vi "624WPI_CameraRead MJPG for Dashboard.vi"(6 "Camera Settings":T2={"fps"=30, "compression"=30, "Image Size"=enum."320x240", "Config Shown"=FALSE}, 7 "USB Cam TCP Port":u16=1180, 8 "Rec Mode":u16(ring) items=["O", "*", "Open Playback Panel"], 9 "Camera IP":string, 10 "Camera Mode":u16(ring) items=["Camera Off", "USB Camera SW", "USB Camera HW", "IP Camera"], 11 "Refnum in":T1) -> (2 "Active":bool, 3 "Refnum out":T1, 4 "FPS":dbl, 5 "Bandwidth (Mbps)":dbl)   [LabVIEW 2016]
uses:
  <vilib>/Rock Robotics/WPI/Camera/WPI_CameraSettings Read MJPG.ctl
  <vilib>/Rock Robotics/WPI/Camera/WPI_CameraImageSize.ctl
  <vilib>/vision/Image Controls.llb/IMAQ Image.ctl
  <vilib>/Rock Robotics/WPI/Dashboard/WPI_DashboardLogging Global.vi
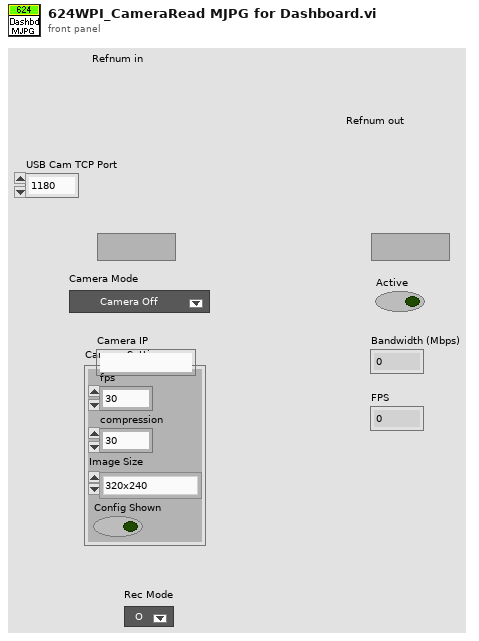
[diagram p1: front panel]
types:
  T1 = typedef "IMAQ Image.ctl" = refnum<image>
  T2 = typedef "WPI_CameraSettings Read MJPG.ctl" = cluster{"fps":i32, "compression":i32, "Image Size":T3, "Config Shown":bool}
  T3 = typedef "WPI_CameraImageSize.ctl" = enum16{"640x480", "320x240", "160x120", "Custom"}
  T4 = typedef "IMAQ AVI2 Refnum.ctl" = refnum<k20>
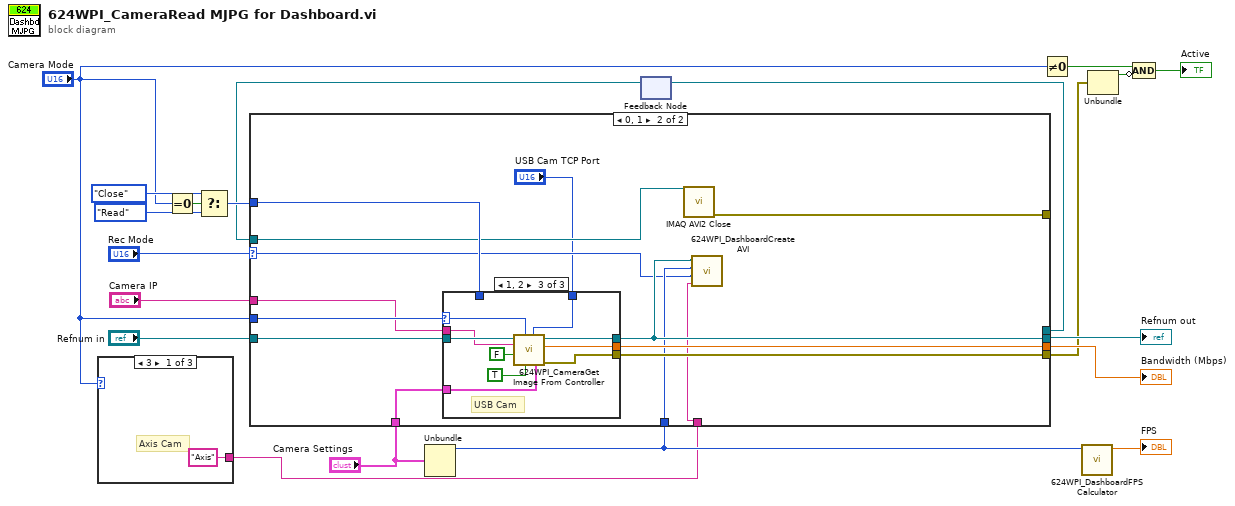
[diagram p0: block diagram]
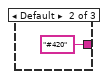
[diagram p2: hidden frame]
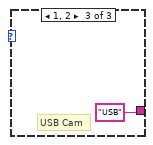
[diagram p3: hidden frame]
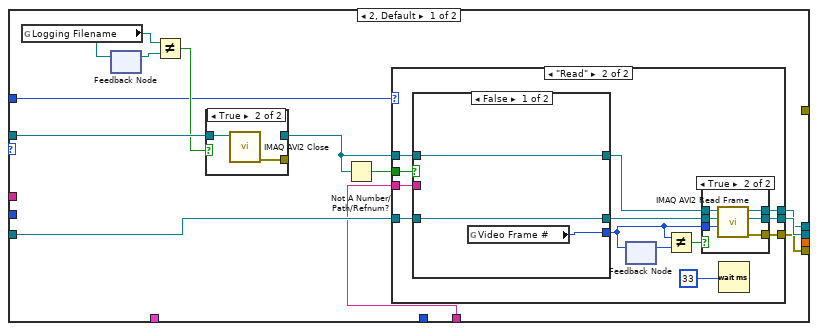
[diagram p4: hidden frame]
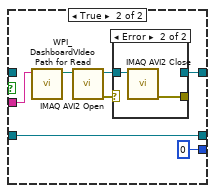
[diagram p7: hidden frame]
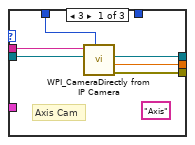
[diagram p10: hidden frame]
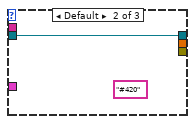
[diagram p11: hidden frame]
diagram:
  n1 = case shown="3" "Camera Mode" {
    tunnel: ["Axis" "#420" "USB"] -> w1
    frame 3 {
      # "Axis Cam"
    }
    frame Default {
    }
    frame 1, 2 {
      # "USB Cam"
    }
  }
  n2 = Equal To 0?(x="Camera Mode") -> (x = 0?=w6:bool)
  n3 = Select(t=enum16{"Read", "Reopen", "Close"}."Close" ("Operation"), s=w6, f=enum16{"Read", "Reopen", "Close"}."Read" ("Operation")) -> (s? t:f=w17:enum16{"Read", "Reopen", "Close"})
  n4 = Unbundle("Camera Settings") -> ("fps"=w4:i32)  [unwired: 3 out]
  n5 = feedback #1() -> (w9:T4)  [unwired: 1 in]
  n6 = case shown="0, 1" "Rec Mode" {
    selector: "Rec Mode" -> [_ w78]
    tunnel: "Camera Settings" -> [_ w88]
    tunnel: w17 -> [w25 w87]
    tunnel: [_ w86] -> w14
    tunnel: [w35 w80] -> w10
    tunnel: "Refnum in" -> [w33 w85]
    tunnel: "Camera IP" -> [_ w77]
    tunnel: w4 -> [_ w79]
    tunnel: w9 -> [w29 w83]
    tunnel: [w32 _] -> w8
    tunnel: [w31 w84] -> w7
    tunnel: [_ w82] -> _
    tunnel: "Camera Mode" -> [_ w81]
    tunnel: w1 -> [w24 w75]
    frame 2, Default {
      n7 = global read "WPI_DashboardLogging Global.vi" "Logging Filename"() -> (w28:path)
      n8 = feedback #2() -> (w27:path)  [unwired: 1 in]
      n9 = feedback-in #2(w28) -> ()
      n10 = Not Equal?(x=w28, y=w27) -> (x != y?=w26:bool)
      n11 = case shown="True" w26 {
        tunnel: [w72 _] -> w30
        tunnel: w29 -> [w72 w74]
        tunnel: [_ w73] -> _
        frame False {
        }
        frame True {
          n12 = call "IMAQ AVI2 Close"("AVI Refnum"=w74) -> ("error out"=w73:errorcluster)  [unwired: 10 in]
        }
      }
      n13 = Not A Number/Path/Refnum?(number/path/refnum=w30) -> (NaN/Path/Refnum?=w34:bool)
      n14 = case shown="\"Read\"" w25 {
        tunnel: [w36 w50] -> w35
        tunnel: w34 -> [_ w49]
        tunnel: w33 -> [w36 w46]
        tunnel: [w37 w45] -> w32
        tunnel: [_ w44] -> w31
        tunnel: w24 -> [_ w43]
        tunnel: w30 -> [w37 w42]
        frame "Close", Default {
        }
        frame "Read" {
          n15 = case shown="False" w49 {
            tunnel: [w61 w66] -> w48
            tunnel: w42 -> [w61 _]
            tunnel: [w60 w68] -> w47
            tunnel: w46 -> [w60 w68]
            tunnel: [w59 0 ("Video Frame #")] -> w39
            tunnel: w43 -> [_ w63]
            frame False {
              n16 = global read "WPI_DashboardLogging Global.vi" "Video Frame #"() -> (w59:i32)
            }
            frame True {
              n17 = call <vilib>:"WPI_DashboardVIdeo Path for Read.vi"("Camera IP"=w63) -> ("Video Path"=w62:path)  [unwired: 10 in]
              n18 = call "IMAQ AVI2 Open"("AVI File Path"=w62) -> ("error out"=w67:errorcluster, "AVI Refnum"=w65:T4)  [unwired: 9 in]
              n19 = case shown="Error" w67 {
                tunnel: [w69 _] -> w66
                tunnel: w65 -> [w69 w71]
                tunnel: [_ w70] -> _
                frame No Error {
                }
                frame Error {
                  n20 = call "IMAQ AVI2 Close"("AVI Refnum"=w71) -> ("error out"=w70:errorcluster)  [unwired: 10 in]
                }
              }
            }
          }
          n21 = feedback #3() -> (w40:i32)  [unwired: 1 in]
          n22 = feedback-in #3(w39) -> ()
          n23 = Not Equal?(x=w39, y=w40) -> (x != y?=w41:bool)
          n24 = case shown="True" w41 {
            tunnel: [w51 w58] -> w50
            tunnel: w48 -> [w52 w57]
            tunnel: w47 -> [w51 w56]
            tunnel: [w52 w55] -> w45
            tunnel: [_ w54] -> w44
            tunnel: w39 -> [_ w53]
            frame False {
            }
            frame True {
              n25 = call "IMAQ AVI2 Read Frame"("Frame Number"=w53, "Image"=w56, "AVI Refnum"=w57) -> ("error out"=w54:errorcluster, "Image Out"=w58:T1, "AVI Refnum (duplicate)"=w55:T4)  [unwired: 6 in]
            }
          }
          n26 = Wait (ms)(milliseconds to wait=33) -> ()  [unwired: 1 out]
        }
      }
    }
    frame 0, 1 {
      n27 = case shown="1, 2" w81 {
        selector: w81 -> [_ _ w98]
        tunnel: w88 -> [_ _ w100]
        tunnel: w87 -> [w89 _ _]
        tunnel: [w93 _ w99] -> w86
        tunnel: w85 -> [w91 w95 w105]
        tunnel: w77 -> [w90 _ w102]
        tunnel: [w94 _ w103] -> w84
        tunnel: [w92 w95 w104] -> w80
        tunnel: "USB Cam TCP Port" -> [_ _ w97]
        frame 3 {
          (unwired) "Axis"
          # "Axis Cam"
          n28 = call <vilib>:"WPI_CameraDirectly from IP Camera.vi"("Operation"=w89, "Image"=w91, "address"=w90) -> ("error out"=w94:errorcluster, "Bandwidth (Mbps)"=w93:dbl, "Image Out"=w92:T1)  [unwired: 6 in]
        }
        frame Default {
          (unwired) "#420"
        }
        frame 1, 2 {
          # "USB Cam"
          n29 = call "624WPI_CameraGet Image From Controller.vi"("Camera Settings"=w100, "port"=w97, "USB"=TRUE, "Camera Mode"=w98, "Close?"=FALSE, "Controller Address"=w102, "Image"=w105) -> ("error out"=w103:errorcluster, "Bandwidth (Mbps)"=w99:dbl, "Image Out"=w104:T1)  [unwired: 2 in]
        }
      }
      n30 = call "IMAQ AVI2 Close"("AVI Refnum"=w83) -> ("error out"=w82:errorcluster)  [unwired: 10 in]
      n31 = call "624WPI_DashboardCreate AVI.vi"("Camera IP"=w75, "Recording"=w78, "frames per seconds"=w79, "Image"=w80) -> ()  [unwired: 8 in]
    }
  }
  "Bandwidth (Mbps)" <- w14
  "Refnum out" <- w10
  n32 = feedback-in #1(w8) -> ()
  n33 = Not Equal To 0?(x="Camera Mode") -> (x != 0?=w5:bool)
  n34 = call "624WPI_DashboardFPS Calculator.vi"("Average Count"=w4) -> ("fps"=→"FPS":dbl)  [unwired: 10 in]
  n35 = Unbundle(w7) -> ("status"=w18:bool)  [unwired: 2 out]
  n36 = Compound Arithmetic op=AND(w5, invert w18) -> (→"Active":bool)
